vi "Request Enqueuer by Name.vi"(8 "error in (no error)":errorcluster, 10 "Enqueuer Name":string, 11 "Enqueuer Look Up Table in":refnum<class "Enqueuer Look Up Table.lvclass">) -> (0 "error out":errorcluster, 1 "Found?":bool, 2 "Enqueuer":refnum<class "Message Enqueuer.lvclass">, 3 "Enqueuer Look Up Table out":refnum<class "Enqueuer Look Up Table.lvclass">)   [LabVIEW 2016, in "Stream Mediator.lvlib" / "Enqueuer Look Up Table.lvclass"]
doc: "--\nCopyright © 2017 Composed SystemsI All rights reserved.\n\nAuthor: Jon McBee <jon.mcbee@composed.io>\n\nThis library is provided \"AS IS\" ,WITHOUT WARRANTIES OR\nCONDITIONS OF ANY KIND, either express or implied.\n\nComposed Systems -- composed.io\n\nStream 0.0.1.1\nJon McBee - Composed Systems\nCopyright (c) 2017, Composed Systems"
uses:
  <userlib>/Composed Systems/Stream/Mediator/Classes/Enqueuer Look Up Table/Enqueuer Look Up Table.lvclass
  C:/Program Files (x86)/National Instruments/LabVIEW 2016/user.lib/Composed Systems/Stream/Look Up Table/Look Up Table/Look Up Table.lvclass
  <vilib>/ActorFramework/Message Enqueuer/Message Enqueuer.lvclass
  <userlib>/Composed Systems/Stream/Look Up Table/Look Up Table/Look Up Table.lvclass
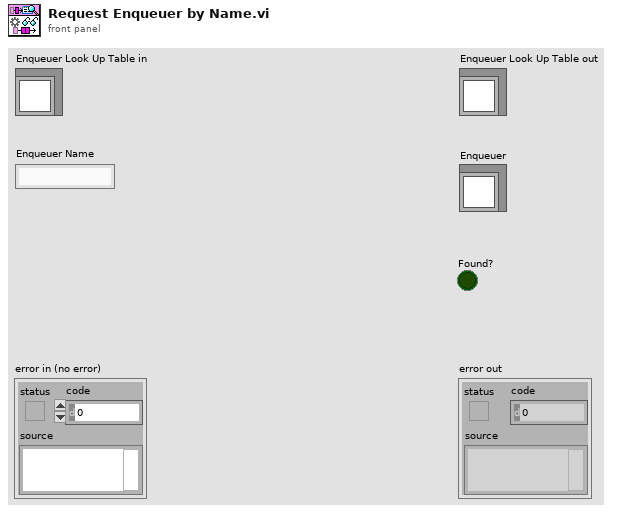
[diagram p1: front panel]
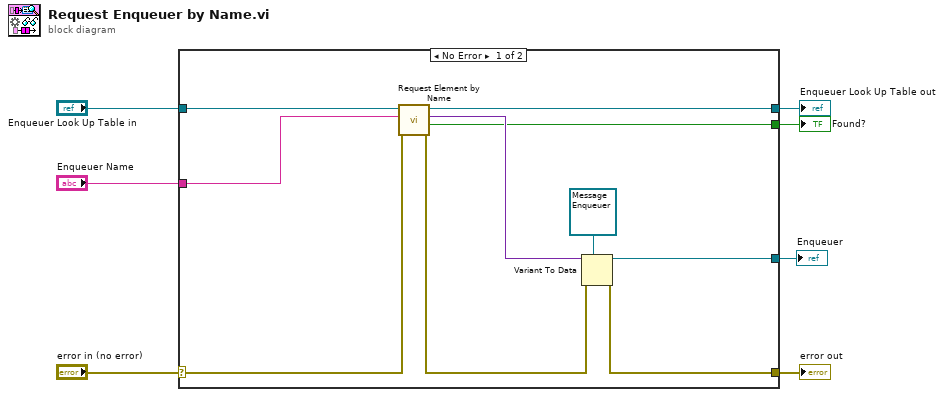
[diagram p0: block diagram]
diagram:
  n1 = case shown="No Error" "error in (no error)" {
    selector: "error in (no error)" -> [w14 w19]
    tunnel: [w17 w19] -> w6
    tunnel: [w10 w18] -> w4
    tunnel: "Enqueuer Look Up Table in" -> [w11 w18]
    tunnel: "Enqueuer Name" -> [w12 _]
    tunnel: [w8 _] -> w2
    tunnel: [w15 _] -> w1
    frame No Error {
      n2 = call <userlib>:"Request Element by Name.vi"("error in (no error)"=w14, "Name"=w12, "Look Up Table in"=w11) -> ("error out"=w13:errorcluster, "Found?"=w8:bool, "Element"=w9:variant, "Look Up Table out"=w10:refnum<class "Enqueuer Look Up Table.lvclass">)  [unwired: 5 in]
      n3 = Variant To Data(error in=w13, type=refnum<class "Message Enqueuer.lvclass"> refnum ("Actor's Enqueuer"), Variant=w9) -> (data=w15:refnum<class "Message Enqueuer.lvclass">, error out=w17:errorcluster)
    }
    frame Error {
    }
  }
  "error out" <- w6
  "Enqueuer Look Up Table out" <- w4
  "Found?" <- w2
  "Enqueuer" <- w1
